vi "test_magnitude.vi"() -> ()   [LabVIEW 2013]
uses:
  <vilib>/rvi/FXPMathLib/FxpSub/XNode/nifxpmath_Sub.xnode
  <vilib>/rvi/FXPMathLib/sim/FxpSim.dll
panel:
  out "Waveform Graph 4":dbl[](graph)
  out "Waveform Graph 2":dbl[][](graph)
  out "size(s)":i32[](array[numeric])
  out "I":dbl[](array[numeric])
  out "Waveform Graph":dbl[][](graph)
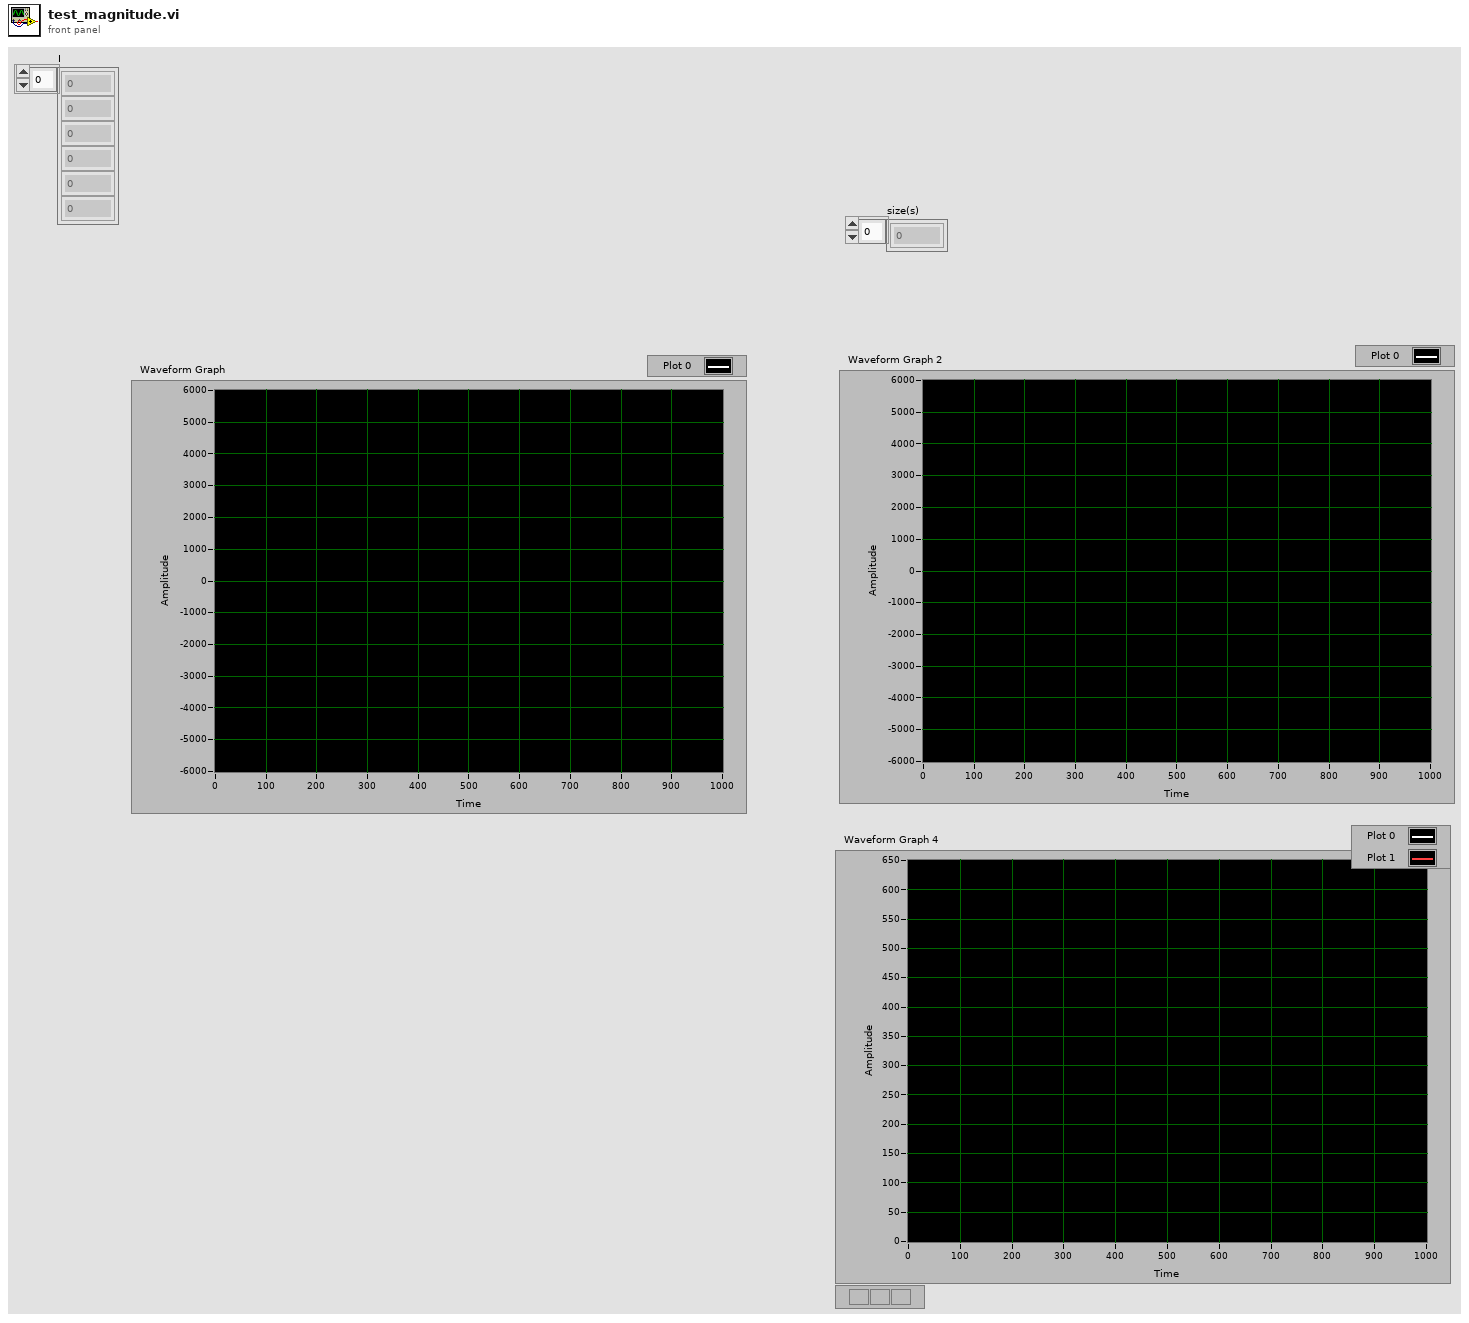
[diagram p1: front panel]
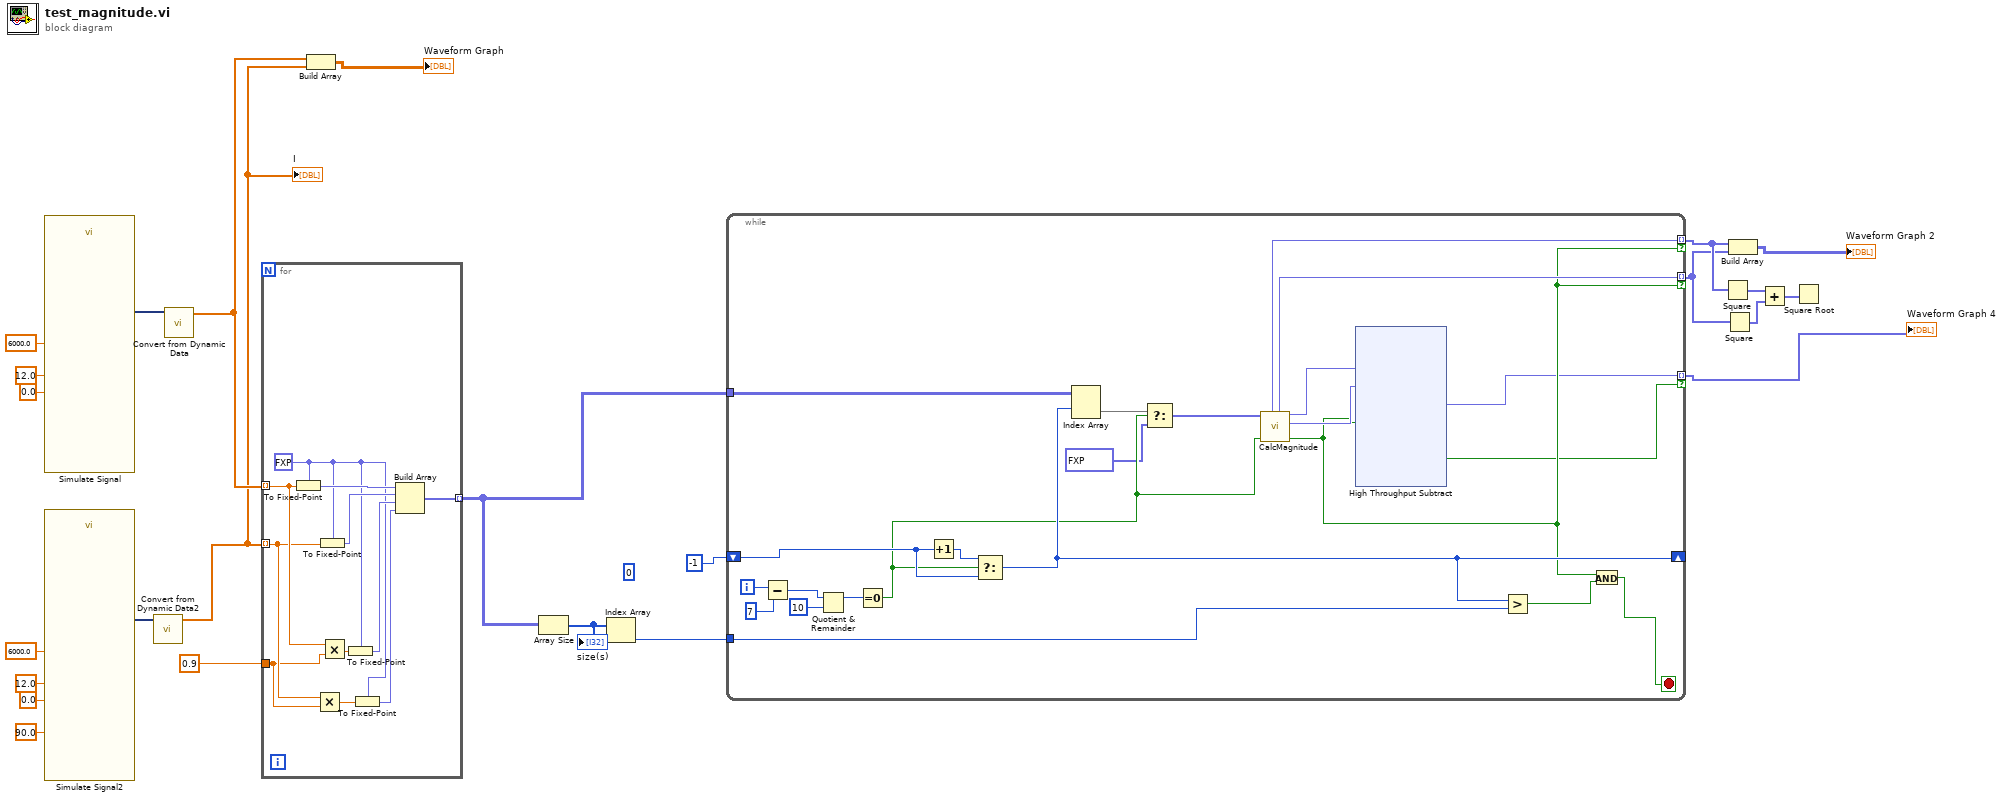
[diagram p0: block diagram]
diagram:
  (unwired) 0
  n1 = call "Simulate Signal"("Frequency"=12.0, "Amplitude"=6000.0, "Noise amplitude"=0.0) -> ("Sine with Uniform Noise"=w24:dynamicdata)  [unwired: 11 in, 1 out]
  n2 = call "Simulate Signal2"("Frequency"=12.0, "Amplitude"=6000.0, "Phase"=90.0, "Noise amplitude"=0.0) -> ("Sine with Uniform Noise"=w22:dynamicdata)  [unwired: 10 in, 1 out]
  n3 = call "Convert from Dynamic Data2"("Dynamic Data Type"=w22) -> ("Array"=w20:dbl[])  [unwired: 3 in]
  "I" <- w20
  n4 = call "Convert from Dynamic Data"("Dynamic Data Type"=w24) -> ("Array"=w21:dbl[])  [unwired: 3 in]
  n5 = for {
    tunnel: w20 -> [w31] mode=indexing
    tunnel: w21 -> [w32] mode=indexing
    tunnel: [w33] -> w12 mode=indexing
    tunnel: 0.9 ("Phase") -> [w30]
    w25 = fxp<+/-,16,14> 0.0 ("f")
    n6 = To Fixed-Point(fixed-point type=w25, number=w32) -> (fixed-point=w35:fxp<+/-,16,14>)
    n7 = Multiply(x=w31, y=w30) -> (x*y=w29:dbl)
    n8 = To Fixed-Point(fixed-point type=w25, number=w31) -> (fixed-point=w34:fxp<+/-,16,14>)
    n9 = Multiply(x=w32, y=w30) -> (x*y=w27:dbl)
    n10 = To Fixed-Point(fixed-point type=w25, number=w27) -> (fixed-point=w26:fxp<+/-,16,14>)
    n11 = To Fixed-Point(fixed-point type=w25, number=w29) -> (fixed-point=w28:fxp<+/-,16,14>)
    n12 = Build Array(w35, w34, w26, w28) -> (w33:fxp<+/-,16,14>[])
  }
  n13 = Build Array(w21, w20) -> (→"Waveform Graph":dbl[][])
  n14 = Array Size(array=w12) -> (size(s)=w14:i32[])
  "size(s)" <- w14
  n15 = Index Array(array=w14) -> (element=w11:i32)  [unwired: 1 in]
  n16 = while {
    tunnel: w12 -> [w52]
    shift-right: [w54] -> _
    shift-left: -1 ("y") -> [w55]
    tunnel: [w42] -> w9 mode=indexing if=w38
    tunnel: [w36] -> w2 mode=indexing if=w37
    tunnel: w11 -> [w43]
    tunnel: [w41] -> w8 mode=indexing if=w38
    i -> [w51]
    stop <- w47 stop-if-true
    n17 = Subtract(x=w51, y=7) -> (x-y=w49:i32)
    n18 = Quotient & Remainder(x=w49, y=10) -> (x-y*floor(x/y)=w57:i32)  [unwired: 1 out]
    n19 = Equal To 0?(x=w57) -> (x = 0?=w45:bool)
    n20 = Increment(x=w55) -> (x+1=w56:i32)
    n21 = Select(t=w56, s=w45, f=w55) -> (s? t:f=w54:i32)
    n22 = Index Array(array=w52, index (row)=w54) -> (element=w53:fxp<+/-,16,14>[])  [unwired: 1 in]
    n23 = Select(t=w53, s=w45, f=fxp<+/-,16,14>[] [0.0, 0.0, 0.0, 0.0] ("Data in")) -> (s? t:f=w46:fxp<+/-,16,14>[])
    n24 = call "CalcMagnitude.vi"("input valid"=w45, "Data in"=w46) -> ("output valid"=w38:bool, "Amp1"=w39:fxp<+,16,14>, "Amp0"=w40:fxp<+,16,14>, "Q0 in"=w41:fxp<+/-,16,14>, "I0 in"=w42:fxp<+/-,16,14>)  [unwired: 5 in]
    n25 = xnode "High Throughput Subtract"("x"=w40, "y"=w39, "input valid"=w38) -> ("x-y"=w36:fxp<+/-,17,15>, "output valid"=w37:bool)  [unwired: 1 in, 1 out]
    n26 = Greater?(x=w54, y=w43) -> (0:w48:bool)
    n27 = And(x=w38, y=w48) -> (x .and. y?=w47:bool)
  }
  "Waveform Graph 4" <- w2
  n28 = Square(x=w9) -> (x^2=w5:fxp<+,31,27>[])
  n29 = Square(x=w8) -> (x^2=w7:fxp<+,31,27>[])
  n30 = Build Array(w9, w8) -> (→"Waveform Graph 2":fxp<+/-,16,14>[][])
  n31 = Add(x=w5, y=w7) -> (x+y=w6:fxp<+,32,28>[])
  n32 = Square Root(x=w6) -> ()  [unwired: 1 out]
